vi "Check for Discrete Input Mapping Conflicts.vi"(8 "error in (no error)":errorcluster, 11 "Coiil Group Ref in":T1 format="%.0x") -> (0 "error out":errorcluster, 1 "Conflicts?":bool, 2 "Conflicts":T2(array[cluster]), 3 "Coil Group Ref out":T1 format="%.0x")   [LabVIEW 2015, in "Modbus Master System Explorer.lvlib"]
uses:
  Modbus Master System Explorer.lvlib
  <vilib>/NI Veristand/Custom Device API/Custom Device Item Ref.ctl
  SubVIs/Modbus Type.ctl
  <vilib>/NI VeriStand/Custom Device API/Custom Device API.lvlib
  Shared/Modbus Master Shared.lvlib
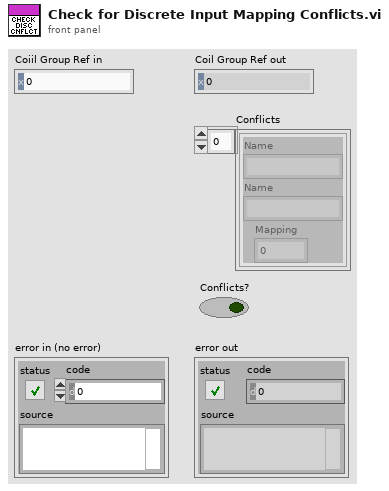
[diagram p1: front panel]
types:
  T1 = typedef "Custom Device API.lvlib/Custom Device Item Ref.ctl" = u64
  T2 = cluster{"Name":string, "Name":string, "Mapping":u16}[]
  T3 = typedef "Modbus Master Shared.lvlib/Modbus Type.ctl" = enum16{"Coil", "Discrete Input", "Holding Register", "Input Register"}
  T4 = typedef "Custom Device API.lvlib/Custom Device Item Info.ctl" = cluster{"Name":string, "Is Channel":bool, "GUID":string, "Is Waveform":bool}
  T5 = cluster{"Name":string, "Name":string, "Mapping":u16}
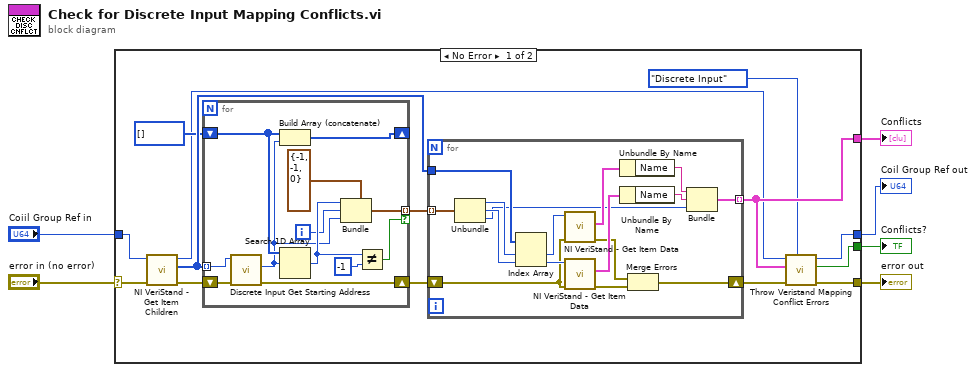
[diagram p0: block diagram]
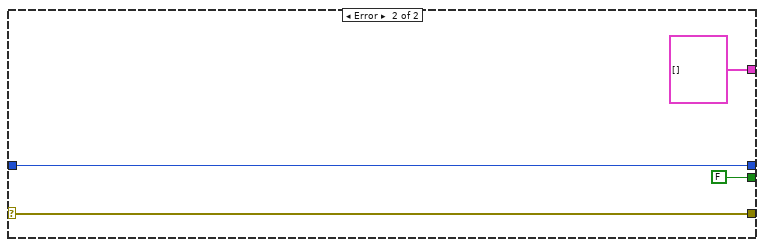
[diagram p2: hidden frame]
diagram:
  n1 = case shown="No Error" "error in (no error)" {
    selector: "error in (no error)" -> [w14 w50]
    tunnel: [w20 T2 []] -> w6
    tunnel: "Coiil Group Ref in" -> [w16 w51]
    tunnel: [w15 w50] -> w4
    tunnel: [w8 w51] -> w2
    tunnel: [w7 FALSE ("Conflicts?")] -> w1
    frame No Error {
      n2 = call <vilib>:"NI VeriStand - Get Item Children.vi"("error in (no error)"=w14, "Item Ref in"=w16) -> ("error out"=w13:errorcluster, "Child Refs"=w19:T1[], "Item Ref out"=w10:T1)  [unwired: 6 in, 1 out]
      n3 = for {
        tunnel: w19 -> [w48] mode=indexing
        shift-right: [w47] -> _
        shift-left: u16[] [] ("Starting Address") -> [w46]
        tunnel: [w43] -> w18 mode=indexing if=w42
        shift-right: [w37] -> w12
        shift-left: w13 -> [w38]
        i -> [w40]
        n4 = call "Discrete Input Get Starting Address.vi"("error in (no error)"=w38, "Item Ref in"=w48) -> ("error out"=w37:errorcluster, "Starting Address"=w39:u16)  [unwired: 7 in, 1 out]
        n5 = Build Array (concatenate)(w46, w39) -> (w47:u16[])
        n6 = Search 1D Array(1D array=w46, element=w39) -> (index of element=w41:i32)  [unwired: 1 in]
        n7 = Bundle(cluster=cluster{"y":i32, "y 2":i32, "Mapping":u16} {"y"=-1, "y 2"=-1, "Mapping"=0} ("Conflicting Indices"), "y"=w41, "y 2"=w40, "Mapping"=w39) -> (w43:cluster{"y":i32, "y 2":i32, "Mapping":u16})
        n8 = Not Equal?(x=w41, y=-1) -> (x != y?=w42:bool)
      }
      n9 = for {
        tunnel: w18 -> [w36] mode=indexing
        tunnel: w19 -> [w35]
        tunnel: [w26] -> w20 mode=indexing
        shift-right: [w21] -> w11
        shift-left: w12 -> [w24]
        n10 = Unbundle(w36) -> ("y"=w34:i32, "y 2"=w33:i32, "Mapping"=w25:u16)
        n11 = Index Array(array=w35, index #1=w34, index #2=w33) -> (element #1=w32:T1, element #2=w31:T1)
        n12 = call <vilib>:"NI VeriStand - Get Item Data.vi"("error in (no error)"=w24, "Item Ref in"=w32) -> ("error out"=w23:errorcluster, "Item Info"=w30:T4)  [unwired: 8 out]
        n13 = call <vilib>:"NI VeriStand - Get Item Data.vi"("error in (no error)"=w24, "Item Ref in"=w31) -> ("error out"=w22:errorcluster, "Item Info"=w29:T4)  [unwired: 8 out]
        n14 = Unbundle By Name(w30) -> ("Name"=w28:string)
        n15 = Unbundle By Name(w29) -> ("Name"=w27:string)
        n16 = Merge Errors(w23, w22) -> (w21:errorcluster)
        n17 = Bundle("Name"=w28, "Name"=w27, "Mapping"=w25) -> (w26:T5)  [unwired: 1 in]
      }
      n18 = call "Throw Veristand Mapping Conflict Errors.vi"("Type"=Modbus_Type."Discrete Input", "error in (no error)"=w11, "Conflicts In"=w20, "Item Ref in"=w10) -> ("error out"=w15:errorcluster, "Conflicts?"=w7:bool, "Node Ref out"=w8:T1)  [unwired: 5 in]
    }
    frame Error {
    }
  }
  "Conflicts?" <- w1
  "Conflicts" <- w6
  "Coil Group Ref out" <- w2
  "error out" <- w4
